vi "Test Pressure Calibration.vi"() -> ()   [LabVIEW 2012]
uses:
  Builder/P Cal Builder.lvclass
  <vilib>/Platform/TimedLoop/XDataNode/timing_clust.ctl
  <vilib>/Platform/TimedLoop/XDataNode/nitl_modes.ctl
  <vilib>/Platform/TimedLoop/XDataNode/wakeup.ctl
  Builder/P Cal Builder.lvclass/P Cal Builder.ctl
  Reusable/Sequence/SEQ/SEQ.lvclass
  Builder/Accessors/Write Pressure.vi
  Builder/Accessors/Write Time.vi
  Builder/Accessors/Write WaitAtMin.vi
  <vilib>/Platform/TimedLoop/XDataNode/XDataNode.xnode
  <vilib>/Platform/TimedLoop/XDataNode/XDNodeRunTimeDep.lvlib
panel:
  in  "stop":bool
  out "seqMsg 2":string[](array[string])=["1:09:27 PM\tValve to oxygen changed to TRUE.", "1:09:27 PM\tO2 flow set to 500.000000.", "1:09:32 PM\tMax orifice flow recorded.   Flow was 248.806366.", "1:09:42 PM\tStandard wait time elapsed.", "1:09:54 PM\tStandard wait time elapsed.", "1:09:55 PM\tLaser RMS stable in every cell. RSE Values: 0.000000\t0.000000\r\n", "1:09:55 PM\tSpeaker position changed to TRUE.", "1:09:55 PM\tO2 flow set to 248.806366.", "1:10:01 PM\tOzone stable in every cell.  Begin collecting data. RSE Values: 0.043430\t0.043108\t0.043108\t0.043537\t0.043537\t0.047428\t0.047428\t0.043882\t0.043882\t0.044978\t0.044978\t0.043616\t0.043616\t0.042956\r\n", "1:10:21 PM\tCollection step complete.", "1:10:21 PM\tO2 flow set to 186.604774.", "1:10:27 PM\tOzone stable in every cell.  Begin collecting data. RSE Values: 0.049616\t0.048562\t0.048562\t0.048143\t0.048143\t0.048496\t0.048678\t0.048678\t0.047656\t0.047656\t0.046716\t0.046716\t0.046716\r\n", "1:10:47 PM\tCollection step complete.", "1:10:47 PM\tO2 flow set to 124.403183.", "1:10:53 PM\tOzone stable in every cell.  Begin collecting data. RSE Values: 0.045074\t0.045269\t0.045269\t0.045371\t0.045371\t0.046657\t0.046657\t0.044803\t0.044803\t0.046626\t0.046626\t0.044248\t0.044248\t0.044248\r\n", "1:11:13 PM\tCollection step complete.", "1:11:13 PM\tO2 flow set to 62.201591.", "1:11:19 PM\tOzone stable in every cell.  Begin collecting data. RSE Values: 0.047075\t0.046939\t0.046939\t0.049594\t0.049594\t0.046739\t0.046655\t0.046655\t0.046655\t0.048990\t0.048989\t0.048989\t0.048989\r\n", "1:11:39 PM\tCollection step complete.", "1:11:39 PM\tData displayed!", "1:11:39 PM\tSpeaker position changed to FALSE.", "1:11:39 PM\tValve to oxygen changed to FALSE.", "1:11:39 PM\tO2 flow set to 0.000000.", "1:11:49 PM\tStandard wait time elapsed.", "1:12:02 PM\tStandard wait time elapsed."] caption="Messages"
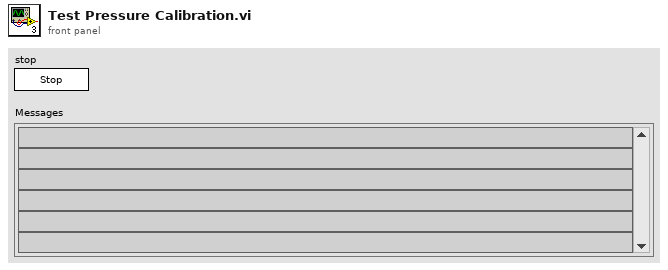
[diagram p1: front panel]
types:
  T1 = typedef "XDNodeRunTimeDep.lvlib/timing_clust.ctl" = cluster{"Expected End [f-1]":u64, "Actual End [f-1]":u64, "Finished Late? [f-1]":bool, "Expected End [i-1]":u64, "Actual End [i-1]":u64, "Finished Late? [i-1]":bool, "Expected Start [i]":u64, "Actual Start [i]":u64, "Expected Start [f]":u64, "Actual Start [f]":u64, "Source Name":string, "Structure Name":string, "Period":i64, "Deadline":i64, "Offset":i64, "Start":i64, "Priority":i32, "Timeout":i32, "Mode":T2, "Wakeup Reason":T3, "Error":errorcluster, "Source Type":string, "Secondary Source Type":string, "Global End Time":u64, "Global Start Time":u64, "Frame Duration":u64, "Iteration Duration":u64, "Assigned CPU":i32, "I/O Scan Engine Mode":u32}
  T2 = typedef "XDNodeRunTimeDep.lvlib/nitl_modes.ctl" = enum32{"No Change", "Process missed periods, maintain original phase", "Discard missed periods, maintain original phase", "Process missed periods, ignore original phase", "Discard missed periods, ignore original phase"}
  T3 = typedef "XDNodeRunTimeDep.lvlib/wakeup.ctl" = enum32{"Normal", "Aborted", "Asynchronous wakeup", "Timing source error", "Timed loop error", "Timeout"}
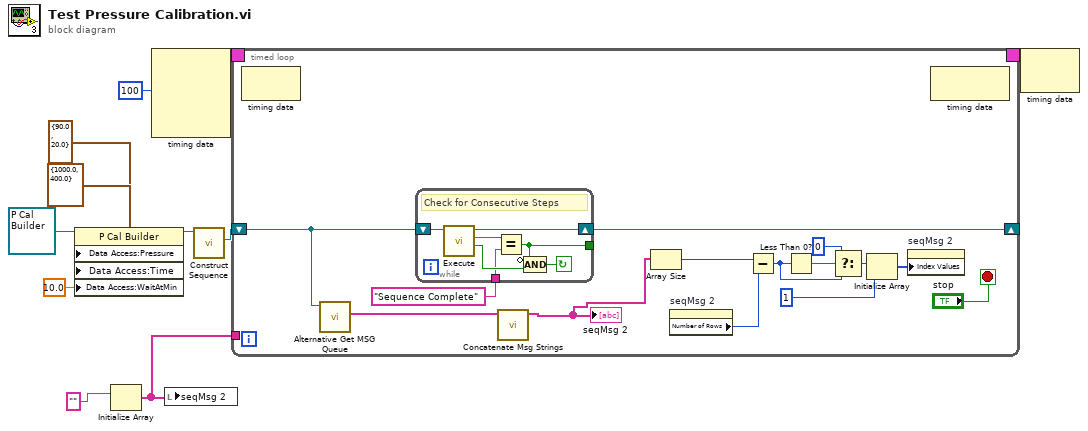
[diagram p0: block diagram]
diagram:
  n1 = property class="P Cal Builder"(reference=refnum<class "P Cal Builder.lvclass"> refnum ("P Cal Builder"), "Data Access:Pressure"=cluster{"Start":dbl, "Final":dbl} {"Start"=1000.0, "Final"=400.0} ("Pressure"), "Data Access:Time"=cluster{"Descent":dbl, "Ascent":dbl} {"Descent"=90.0, "Ascent"=20.0} ("Time"), "Data Access:WaitAtMin"=10.0 ("WaitAtMin")) -> (reference out=w8:refnum<class "P Cal Builder.lvclass">)  [unwired: 1 in, 1 out]
  n2 = Initialize Array("") -> (w4:string[])  [unwired: 1 in]
  n3 = node-c288(i64 100 ("Period")) -> (w3:T1)  [unwired: 3 in]
  n4 = local write "seqMsg 2"(w4) -> ()
  n5 = call-dynamic "Construct Sequence.vi"("P Cal Builder in"=w8) -> ("New Sequence"=w7:refnum<class "SEQ.lvclass">)  [unwired: 8 in, 2 out]
  n6 = timed-loop {
    shift-right: [w25] -> _
    shift-left: w7 -> [w24]
    tunnel: w4 -> [_]
    timing: w3 -> [_]
    timing-out: [_] -> w2
    stop <- "stop" stop-if-true
    n7 = node-c288() -> ()  [unwired: 1 in, 1 out]
    n8 = call "Alternative Get MSG Queue.vi"("SEQ in"=w24) -> ("seqMsg"=w22:string[])  [unwired: 9 in, 1 out]
    n9 = while {
      shift-right: [w33] -> w25
      shift-left: w24 -> [w34]
      tunnel: [w30] -> _
      tunnel: "Sequence Complete" ("t") -> [w28]
      stop <- w31 continue-if-true
      # "Check for Consecutive Steps"
      n10 = call-dynamic "Execute.vi"("SEQ in"=w34) -> ("Next Step?"=w29:bool, "MSG"=w32:string, "SEQ out"=w33:refnum<class "SEQ.lvclass">)  [unwired: 7 in, 1 out]
      n11 = Equal?(x=w32, y=w28) -> (x = y?=w30:bool)
      n12 = Compound Arithmetic op=AND(invert w30, w29) -> (w31:bool)
    }
    n13 = call "Concatenate Msg Strings.vi"("StringsIn"=w22) -> ("StringsOut"=w13:string[])  [unwired: 10 in]
    "seqMsg 2" <- w13
    n14 = Array Size(array=w13) -> (size(s)=w19:i32)
    n15 = property on="seqMsg 2" class="Arr (strict)"() -> ("Number of Rows"=w20:u32)  [unwired: 2 in, 2 out]
    n16 = Subtract(x=w19, y=w20) -> (x-y=w16:u32)
    n17 = Less Than 0?(x=w16) -> (x < 0?=w17:bool)
    n18 = Select(t=u32 0, s=w17, f=w16) -> (s? t:f=w14:u32)
    n19 = Initialize Array(w14, 1 ("dimension size")) -> (w21:u32[])
    n20 = property on="seqMsg 2" class="Arr (strict)"("Index Values"=w21) -> ()  [unwired: 2 in, 2 out]
    n21 = node-c288() -> ()  [unwired: 1 in, 1 out]
  }
  n22 = node-c288(w2) -> ()  [unwired: 1 out]
